vi "SpectralSpread (SubVI).vi"(6 "Frequency Array":dbl[](array[numeric]), 9 "Positve Half of FFT with 0Hz and Nyquist":dbl[](array[numeric]), 10 "Sum of FFT Mags":dbl, 11 "Spectral Centroid":dbl) -> (3 "Spectral Spread":dbl)   [LabVIEW 2015]
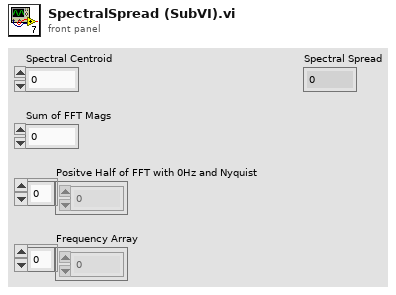
[diagram p1: front panel]
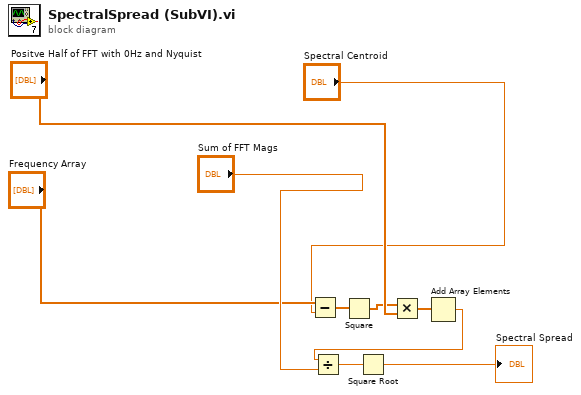
[diagram p0: block diagram]
diagram:
  n1 = Subtract(x="Frequency Array", y="Spectral Centroid") -> (x-y=w3:dbl[])
  n2 = Square(x=w3) -> (x^2=w4:dbl[])
  n3 = Multiply(x=w4, y="Positve Half of FFT with 0Hz and Nyquist") -> (x*y=w5:dbl[])
  n4 = Add Array Elements(numeric array=w5) -> (sum=w6:dbl)
  n5 = Divide(x=w6, y="Sum of FFT Mags") -> (x/y=w8:dbl)
  n6 = Square Root(x=w8) -> (sqrt(x)=→"Spectral Spread":dbl)
